vi "getProcessFolderPath.vi"(8 "error in (no error)":errorcluster) -> (0 "error out":errorcluster, 3 "Process Folder":path)   [LabVIEW 2011]
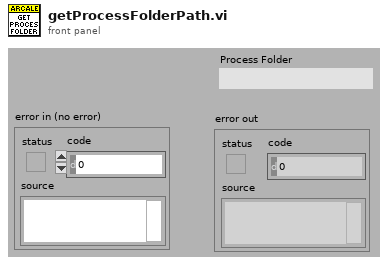
[diagram p1: front panel]
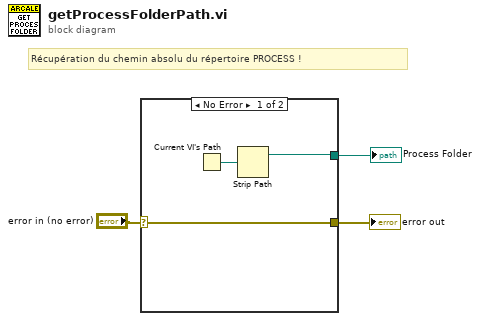
[diagram p0: block diagram]
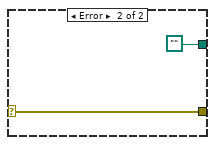
[diagram p2: hidden frame]
diagram:
  # "Récupération du chemin absolu du répertoire PROCESS !"
  n1 = case shown="No Error" "error in (no error)" {
    selector: "error in (no error)" -> [w5 w8]
    tunnel: [w5 w8] -> w3
    tunnel: [w4 path ""] -> w1
    frame No Error {
      n2 = Current VI's Path() -> (path=w6:path)
      n3 = Strip Path(path=w6) -> (stripped path=w4:path)  [unwired: 1 out]
    }
    frame Error {
    }
  }
  "error out" <- w3
  "Process Folder" <- w1
